vi "PP_Profile_Block_Av.vi"() -> ()   [LabVIEW 2016]
uses:
  Controls/File_Selector_Type.ctl
panel:
  in  "Desired Averaging Time (mins)":dbl=1.0
  out "Current File name":path
  in  "stop":bool
  out "Current on file":i32
  out "Number of files":i32
  in  "At Dialog Prompt Post Process":T1
  in  "Results file":path
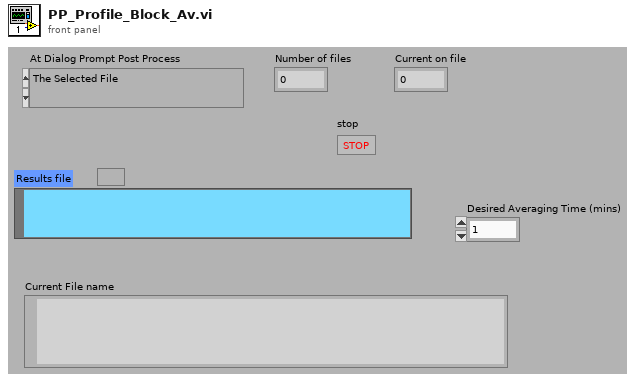
[diagram p1: front panel]
types:
  T1 = typedef "File_Selector_Type.ctl" = enum16{"The Selected File", "The Selected Folder", "Files containing the search string in the selected folder", "All files listed in selected file"}
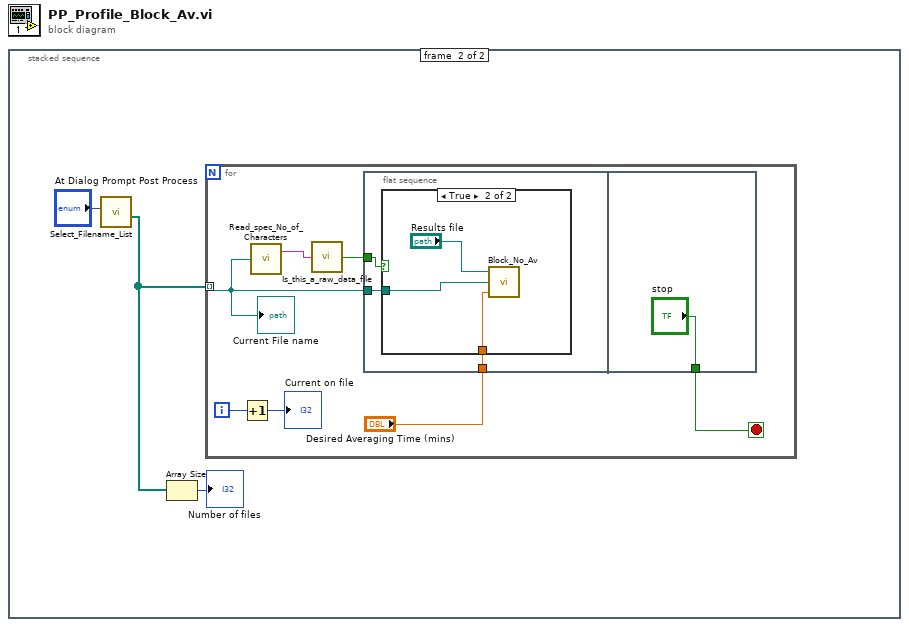
[diagram p0: block diagram]
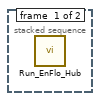
[diagram p2: hidden frame]
diagram:
  n1 = stacked-sequence {
    frame #0 {
      n2 = call "Run_EnFlo_Hub.vi"() -> ()  [unwired: 7 in, 1 out]
    }
    frame #1 {
      n3 = call "Select_Filename_List.vi"("At Dialog Prompt Post Process"="At Dialog Prompt Post Process") -> ("Selected files"=w2:path[])  [unwired: 4 in, 3 out]
      n4 = Array Size(array=w2) -> (size(s)=→"Number of files":i32)
      n5 = for {
        tunnel: w2 -> [w10] mode=indexing
        i -> [w7]
        stop <- w5 stop-if-true
        n6 = Increment(x=w7) -> (x+1=→"Current on file":i32)
        n7 = call "Read_spec_No_of_Characters.vi"("Filename"=w10) -> ("character string"=w9:string)  [unwired: 1 out]
        n8 = call "Is_this_a_raw_data_file.vi"("character string"=w9) -> ("Raw Dat File?"=w8:bool)  [unwired: 2 out]
        n9 = flat-sequence {
          tunnel: w10 -> [w13]
          tunnel: w8 -> [w12]
          tunnel: "Desired Averaging Time (mins)" -> [w11]
          tunnel: ["stop"] -> w5
          frame #0 {
            n10 = case shown="True" w12 {
              tunnel: w13 -> [_ w15]
              tunnel: w11 -> [_ w14]
              frame False {
              }
              frame True {
                n11 = call "Block_No_Av.vi"("Desired Averaging Time (mins)"=w14, "Raw data file"=w15, "Results file"="Results file") -> ()  [unwired: 2 in]
              }
            }
          }
          frame #1 {
          }
        }
        "Current File name" <- w10
      }
    }
  }
